vi "JSONRPC-GetAsType.vi"   [LabVIEW 2014]
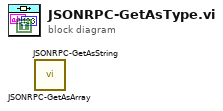
[diagram p0: block diagram]
diagram:
  n1 = call "JSONRPC-GetAsArray.vi"() -> ()  [unwired: 11 in, 1 out]
  n2 = call "JSONRPC-GetAsString.vi"() -> ()  [unwired: 11 in, 1 out]
